vi "Ballard Arinc-429 - Initialization VI.vi"(8 "error in (no error)":errorcluster, 10 "Custom XML":string, 11 "Device Item Ref in":T1 format="%.0x") -> (0 "error out":errorcluster, 3 "Device Item Ref out":T1 format="%.0x")   [LabVIEW 2017, in "Ballard Arinc-429 System Explorer.lvlib"]
uses:
  Ballard Arinc-429 System Explorer.lvlib
  <vilib>/NI Veristand/Custom Device API/Custom Device Item Ref.ctl
  <vilib>/NI Veristand/Custom Device API/Custom Device Channel.ctl
  <vilib>/NI Veristand/Custom Device API/Custom Device Channel Type.ctl
  <vilib>/NI Veristand/Custom Device API/Custom Device Loop Type.ctl
  Shared/Controls and Global/Global.vi
  <vilib>/NI Veristand/Custom Device API/Set Item Property (I32).vi
  <vilib>/NI Veristand/Custom Device API/Custom Device API.lvlib
  Shared/Ballard Arinc-429 Shared.lvlib
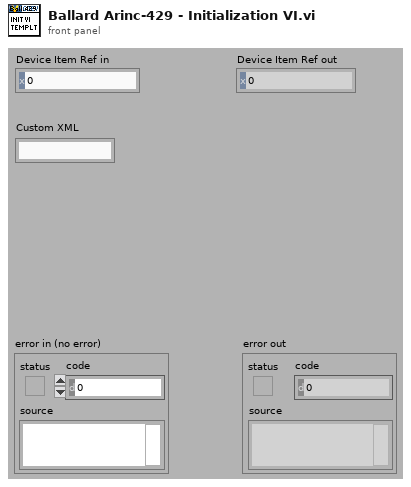
[diagram p1: front panel]
types:
  T1 = typedef "Custom Device API.lvlib/Custom Device Item Ref.ctl" = u64
  T2 = typedef "Custom Device API.lvlib/Custom Device Loop Type.ctl" = enum32{"While Loop", "Timed Loop"}
  T3 = typedef "Custom Device API.lvlib/Custom Device Channel.ctl" = cluster{"Type":T4, "Units":string, "Default Value":dbl, "Faultable":bool, "Scalable":bool}
  T4 = typedef "Custom Device API.lvlib/Custom Device Channel Type.ctl" = enum16{"Input", "Output"}
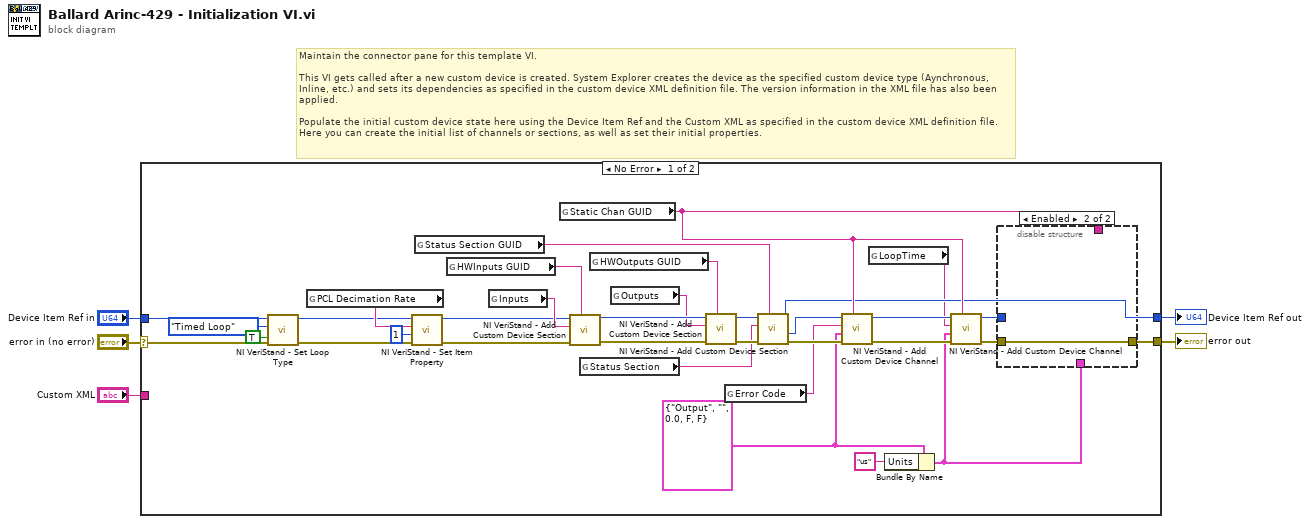
[diagram p0: block diagram]
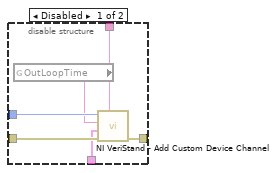
[diagram p2: hidden frame]
diagram:
  # "Maintain the connector pane for this template VI.\n\nThis VI gets called after a new custom device is created. System Explorer creates the device as the specified custom device type (Aynchronous, Inline, etc.) and sets its dependencies as specified in the custom device XML definition file. The version information in the XML file has also been applied.\n\nPopulate the initial custom device state here using the Device Item Ref and the Custom XML as specified in the custom device XML definition file. Here you can create the initial list of channels or sections, as well as set their initial properties."
  n1 = case shown="No Error" "error in (no error)" {
    selector: "error in (no error)" -> [w8 w48]
    tunnel: [w19 w47] -> w4
    tunnel: "Device Item Ref in" -> [w12 w47]
    tunnel: "Custom XML" -> [_ _]
    tunnel: [w20 w48] -> w1
    frame No Error {
      w21 = T3 {"Type"=enum."Output", "Units"="", "Default Value"=0.0, "Faultable"=FALSE, "Scalable"=FALSE} ("Channel")
      n2 = call <vilib>:"NI VeriStand - Set Loop Type.vi"("error in (no error)"=w8, "Use Device Clock (Timed Loops only)"=TRUE, "Loop type"=Custom_Device_Loop_Type."Timed Loop", "Device Ref in"=w12) -> ("error out"=w7:errorcluster, "Device Ref out"=w11:T1)  [unwired: 6 in]
      n3 = global read "Global.vi" "PCL Decimation Rate"() -> (w14:string)
      n4 = call-poly <vilib>:"NI VeriStand - Set Item Property.vi"("error in (no error)"=w7, "Value"=1, "Property Name"=w14, "Item Ref in"=w11) -> ("error out"=w16:errorcluster, "Item Ref out"=w15:T1)  [unwired: 5 in, 1 out]
      n5 = global read "Global.vi" "Status Section GUID"() -> (w29:string)
      n6 = global read "Global.vi" "HWInputs GUID"() -> (w35:string)
      n7 = global read "Global.vi" "Inputs"() -> (w37:string)
      n8 = global read "Global.vi" "Static Chan GUID"() -> (w22:string)
      n9 = call <vilib>:"NI VeriStand - Add Custom Device Section.vi"("GUID (Default Section)"=w35, "error in (no error)"=w16, "Section Name"=w37, "Parent Ref in"=w15) -> ("error out"=w39:errorcluster, "Parent Ref out"=w38:T1)  [unwired: 4 in, 2 out]
      n10 = global read "Global.vi" "Status Section"() -> (w27:string)
      n11 = global read "Global.vi" "HWOutputs GUID"() -> (w34:string)
      n12 = global read "Global.vi" "Outputs"() -> (w36:string)
      n13 = call <vilib>:"NI VeriStand - Add Custom Device Section.vi"("GUID (Default Section)"=w34, "error in (no error)"=w39, "Section Name"=w36, "Parent Ref in"=w38) -> ("error out"=w33:errorcluster, "Parent Ref out"=w32:T1)  [unwired: 4 in, 2 out]
      n14 = global read "Global.vi" "Error Code"() -> (w28:string)
      n15 = call <vilib>:"NI VeriStand - Add Custom Device Section.vi"("GUID (Default Section)"=w29, "error in (no error)"=w33, "Section Name"=w27, "Parent Ref in"=w32) -> ("error out"=w31:errorcluster, "Section Ptr"=w30:T1, "Parent Ref out"=w19:T1)  [unwired: 4 in, 1 out]
      n16 = call <vilib>:"NI VeriStand - Add Custom Device Channel.vi"("GUID (Default Channel)"=w22, "error in (no error)"=w31, "Channel"=w21, "Channel Name"=w28, "Parent Ref in"=w30) -> ("error out"=w26:errorcluster, "Parent Ref out"=w24:T1)  [unwired: 3 in, 2 out]
      n17 = global read "Global.vi" "LoopTime"() -> (w6:string)
      n18 = Bundle By Name(cluster=w21, "Units"="us") -> (w18:T3)
      n19 = call <vilib>:"NI VeriStand - Add Custom Device Channel.vi"("GUID (Default Channel)"=w22, "error in (no error)"=w26, "Channel"=w18, "Channel Name"=w6, "Parent Ref in"=w24) -> ("error out"=w25:errorcluster, "Parent Ref out"=w23:T1)  [unwired: 3 in, 2 out]
      n20 = disable-structure shown="Enabled" {
        disable-tunnel: w25 -> [w45 w46]
        disable-tunnel: w23 -> [w44 _]
        disable-tunnel: w22 -> [w42 _]
        disable-tunnel: [w41 w46] -> w20
        disable-tunnel: w18 -> [w40 _]
        frame Disabled {
          n21 = global read "Global.vi" "OutLoopTime"() -> (w43:string)
          n22 = call <vilib>:"NI VeriStand - Add Custom Device Channel.vi"("GUID (Default Channel)"=w42, "error in (no error)"=w45, "Channel"=w40, "Channel Name"=w43, "Parent Ref in"=w44) -> ("error out"=w41:errorcluster)  [unwired: 3 in, 3 out]
        }
        frame Enabled {
        }
      }
    }
    frame Error {
    }
  }
  "error out" <- w1
  "Device Item Ref out" <- w4
